vi "Periodic Tasks.vi"(8 "error in":errorcluster) -> ()   [LabVIEW 2016]
doc: "This VI runs in parallel to other tasks. It can contain as many user-defined periodic loops as you need. These can carry out PID or other sorts of timed response."
uses:
  Controls/Manual Shooter.ctl
  Controls/Shooter.ctl
  <vilib>/Rock Robotics/WPI/Solenoid/WPI_SolenoidValue.ctl
  <vilib>/Rock Robotics/WPI/DriverStation/WPI_DriverStationRobotMode2.ctl
  Controls/Auto Selector.ctl
  Controls/Gear Intake State.ctl
  Support Code/Change Detect.vi
  Support Code/Change Detect Boolean.vi
  <vilib>/Rock Robotics/WPI/Utilities/WPI_GetSetVariantRefNum.vi
  Robot Global Data.vi
  <vilib>/Rock Robotics/WPI/Solenoid/WPI_SolenoidSetEnum.vi
  <vilib>/Rock Robotics/Network Tables/NT Write Boolean.vi
  Controls/currentState.ctl
panel:
  in  "time to release(ms)":u32=800
  in  "Intake release speed":dbl=-0.5 format="%#_13g"
  in  "Intake gather speed":dbl=1.0 format="%#_13g"
  in  "Turret Deadband":dbl=0.5 format="%#_13g"
  out "Turret Stopped?":bool
  in  "turret error":dbl=4.0 format="%#_13g"
  in  "Turret Limit":dbl=90.0 format="%#_13g"
  out "low pass":dbl
  in  "auto gear on?":bool
  in  "turret reset":bool
  in  "Indexer % M":dbl=0.9 format="%#_13g"
  in  "M - Bot - Boiler":dbl=1450.0 format="%#_13g"
  in  "M - Top - Boiler":dbl=3950.0 format="%#_13g"
  in  "M - Bot - Airship":dbl=1500.0 format="%#_13g"
  in  "M - Top - Airship":dbl=4550.0 format="%#_13g"
  in  "autoGearRate":u32=10
  in  "Bot CPR":dbl=1024.0
  in  "Top CPR":dbl=1.0
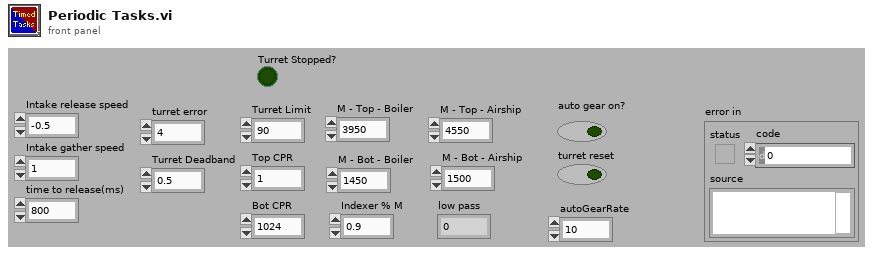
[diagram p1: front panel]
types:
  T1 = typedef "Shooter.ctl" = enum16{"Manual Control", "Get Setpoint", "Check Setpoint"}
  T2 = typedef "Manual Shooter.ctl" = enum16{"init", "Prepare - Airship", "Prepare - Boiler", "Burst mode"}
  T3 = typedef "WPI_RobotDriveDevRef.ctl" = cluster{"DevStatus":errorcluster, "Motors[]":T4[], "Square Inputs":bool, "Max Output":dbl}
  T4 = typedef "WPI_MotorControlDeviceRef.ctl" = cluster{"DeviceStatus":errorcluster, "Type":T5, "PWM":cluster{"PWM Channel":T6, "DeadBand":T7}, "CAN":cluster{"Device Number":u8, "SetOutput VI Ref":variant, "GetOutput VI Ref":variant, "Enable VI Ref":variant, "Disable VI Ref":variant, "Data":variant}, "Invert":bool}
  T5 = typedef "WPI_MotorControlType.ctl" = enum16{"PWM", "CAN"}
  T6 = typedef "FPGA_DIOPWMChannel.ctl" = enum8{"PWM 0", "PWM 1", "PWM 2", "PWM 3", "PWM 4", "PWM 5", "PWM 6", "PWM 7", "PWM 8", "PWM 9", "PWM MXP 0", "PWM MXP 1", "PWM MXP 2", "PWM MXP 3", "PWM MXP 4", "PWM MXP 5", "PWM MXP 6", "PWM MXP 7", "PWM MXP 8", "PWM MXP 9", "Invalid"}
  T7 = typedef "WPI_PWMDeadband.ctl" = cluster{"Name":string, "maxPositivePwm":i32, "minPositivePwm":i32, "centerPwm":i32, "maxNegativePwm":i32, "minNegativePwm":i32, "angularRange":u16}
  T8 = typedef "WPI_SolenoidDevRef.ctl" = cluster{"DevStatus":errorcluster, "Pneumatics Control Module":u8, "Forward Solenoid Channel":T9, "Reverse Solenoid Channel":T9}
  T9 = typedef "WPI_SolenoidChannel.ctl" = enum8{"Solenoid 0", "Solenoid 1", "Solenoid 2", "Solenoid 3", "Solenoid 4", "Solenoid 5", "Solenoid 6", "Solenoid 7", "Invalid"}
  T10 = cluster{"positions[0]":cluster{"x":i32, "y":i32}, "positions[1]":cluster{"x":i32, "y":i32}, "positions[2]":cluster{"x":i32, "y":i32}, "positions[3]":cluster{"x":i32, "y":i32}, "positions[4]":cluster{"x":i32, "y":i32}, "positions[5]":cluster{"x":i32, "y":i32}, "positions[6]":cluster{"x":i32, "y":i32}, "positions[7]":cluster{"x":i32, "y":i32}, "positions[8]":cluster{"x":i32, "y":i32}}
  T11 = cluster{"Buttons[0]":bool, "Buttons[1]":bool, "Buttons[2]":bool, "Buttons[3]":bool, "Buttons[4]":bool, "Buttons[5]":bool, "Buttons[6]":bool, "Buttons[7]":bool, "Buttons[8]":bool}
  T12 = typedef "WPI_SolenoidValue.ctl" = enum16{"Off", "On", "Forward", "Reverse"}
  T13 = typedef "WPI_DriverStationRobotMode2.ctl" = enum16{"Autonomous Disabled", "Autonomous Enabled", "Teleop Disabled", "Teleop Enabled", "Disconnected", "Finish", "Test Disabled", "Test Enabled", "Emergency Stopped"}
  T14 = cluster{"Axes[0]":dbl, "Axes[1]":dbl, "Axes[2]":dbl, "Axes[3]":dbl, "Axes[4]":dbl, "Axes[5]":dbl, "Axes[6]":dbl, "Axes[7]":dbl, "Axes[8]":dbl}
  T15 = typedef "Gear Intake State.ctl" = enum16{"init", "Gather", "Release"}
  T16 = typedef "WPI_DigitalInputDevRef.ctl" = cluster{"DevStatus":errorcluster, "DIO Channel":T17}
  T17 = typedef "FPGA_DIOChannel.ctl" = enum8{"DIO 0", "DIO 1", "DIO 2", "DIO 3", "DIO 4", "DIO 5", "DIO 6", "DIO 7", "DIO 8", "DIO 9", "DIO MXP 0", "DIO MXP 1", "DIO MXP 2", "DIO MXP 3", "DIO MXP 4", "DIO MXP 5", "DIO MXP 6", "DIO MXP 7", "DIO MXP 8", "DIO MXP 9", "DIO MXP 10", "DIO MXP 11", "DIO MXP 12", "DIO MXP 13", "DIO MXP 14", "DIO MXP 15", "SPI Port CS1", "SPI Port CS2", "SPI Port CS3", "SPI Port MISO", "SPI Port MOSI", "Invalid"}
  T18 = typedef "Auto Selector.ctl" = enum16{"Gear + Fuel with Vision", "Gear + Fuel no Vision", "Middle Gear", "Gear - Feeder peg", "Nothing"}
  T19 = cluster{"Top":bool, "Left":bool, "Right":bool, "Bottom":bool}
  T20 = typedef "currentState.ctl" = enum16{"init", "gearUp", "gearDown"}
  T21 = typedef "WPI_CounterDevRef.ctl" = cluster{"DevStatus":errorcluster, "CntIndex":T22}
  T22 = typedef "FPGA_CounterCtrSystemIndex.ctl" = enum8{"Ctr 0", "Ctr 1", "Ctr 2", "Ctr 3", "Ctr 4", "Ctr 5", "Ctr 6", "Ctr 7", "Invalid"}
  T23 = typedef "WPI_EncoderDevRef.ctl" = cluster{"DevStatus":errorcluster, "EncoderIndex":T24, "CounterIndex":T22, "DistancePerCount":dbl, "Decoding Type":T25}
  T24 = typedef "FPGA_EncoderIdx.ctl" = enum8{"Enc 0", "Enc 1", "Enc 2", "Enc 3", "Enc 4", "Enc 5", "Enc 6", "Enc 7", "Invalid"}
  T25 = typedef "WPI_EncoderType.ctl" = enum16{"1x", "2x", "4x"}
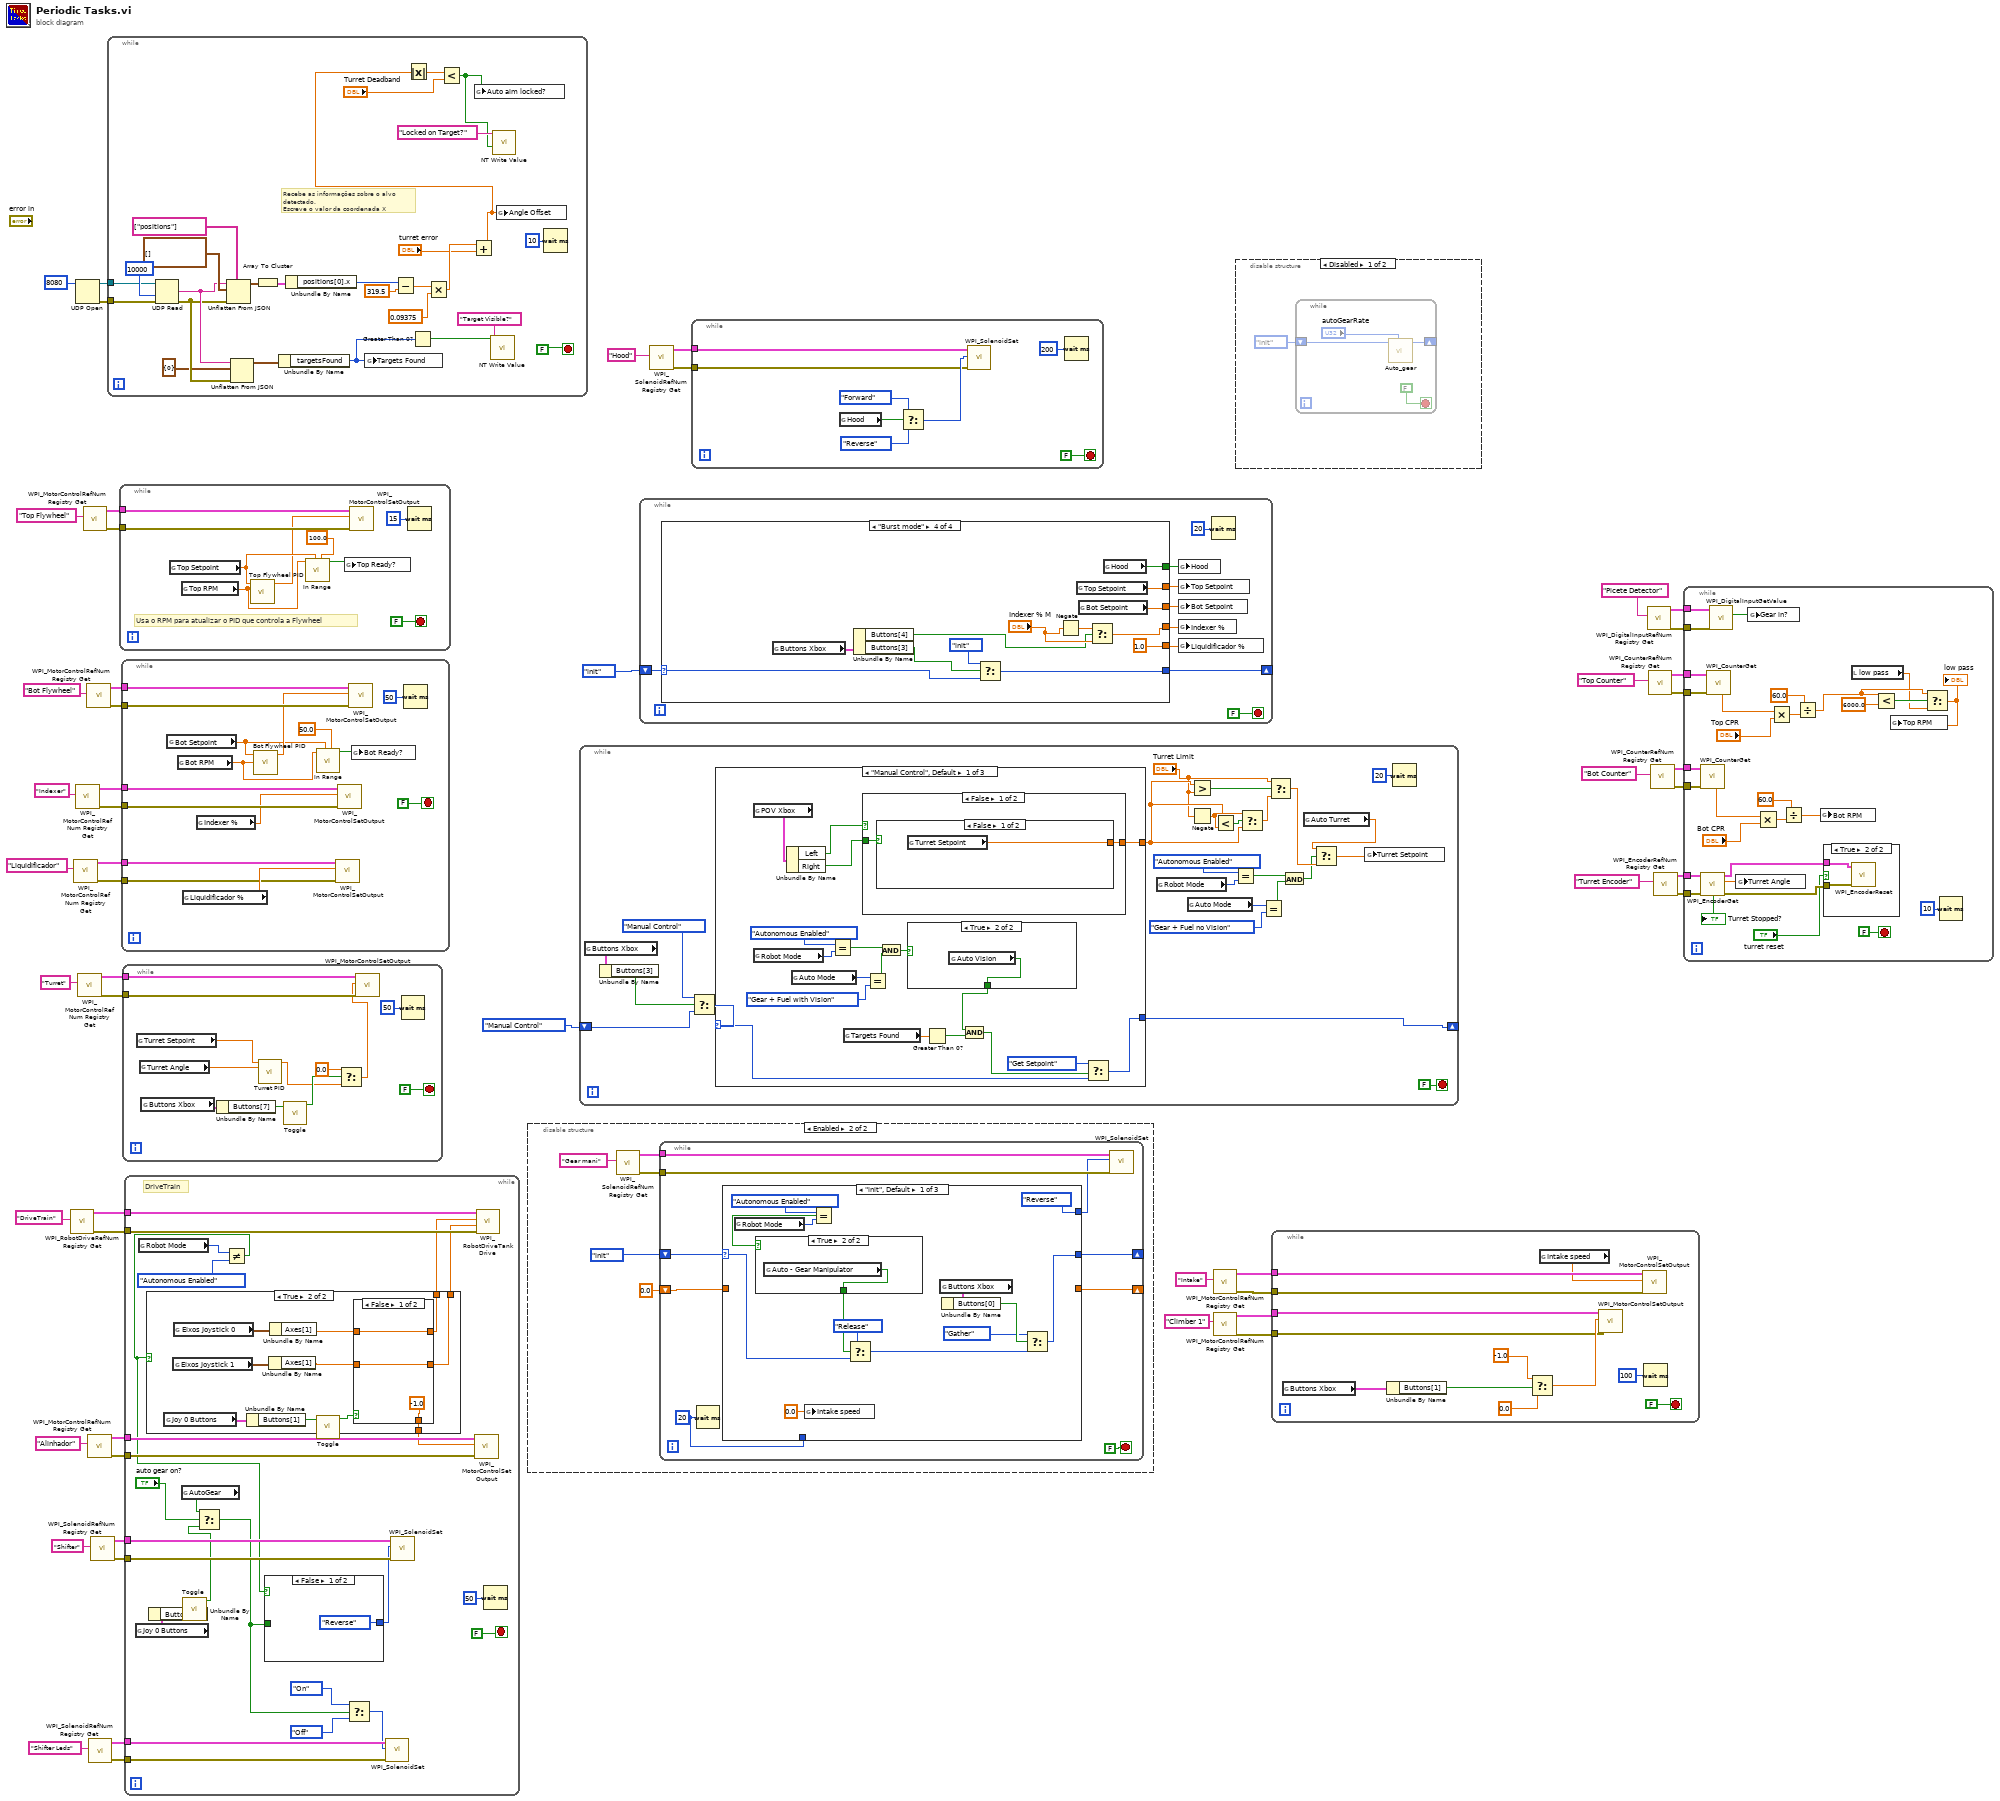
[diagram p0: block diagram]
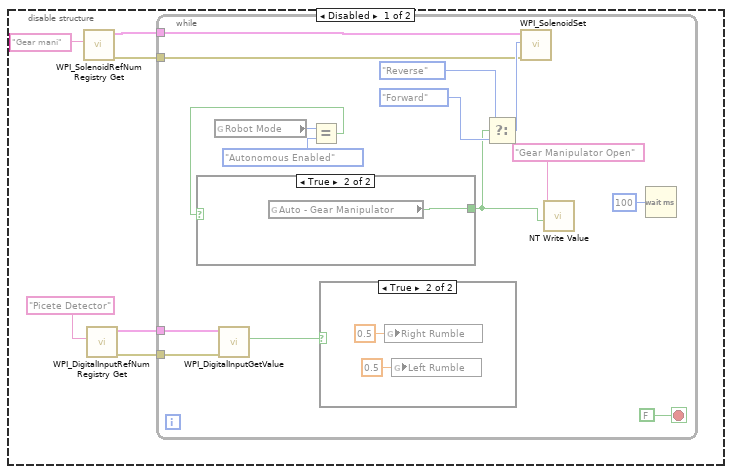
[diagram p2: hidden frame]
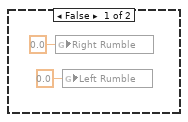
[diagram p3: hidden frame]
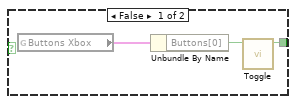
[diagram p4: hidden frame]
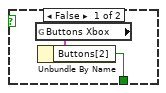
[diagram p5: hidden frame]
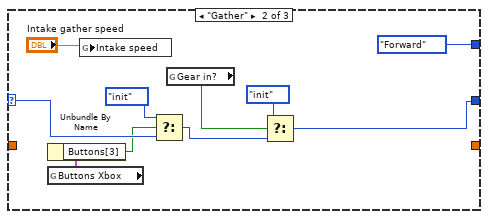
[diagram p6: hidden frame]
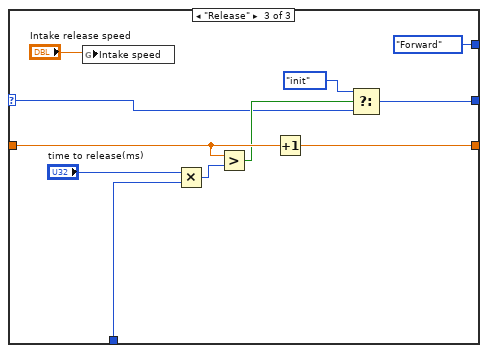
[diagram p7: hidden frame]
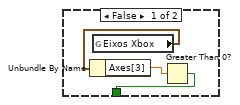
[diagram p9: hidden frame]
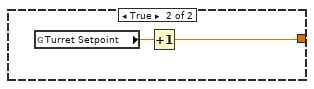
[diagram p10: hidden frame]
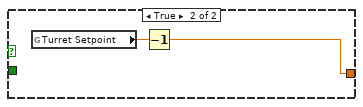
[diagram p11: hidden frame]
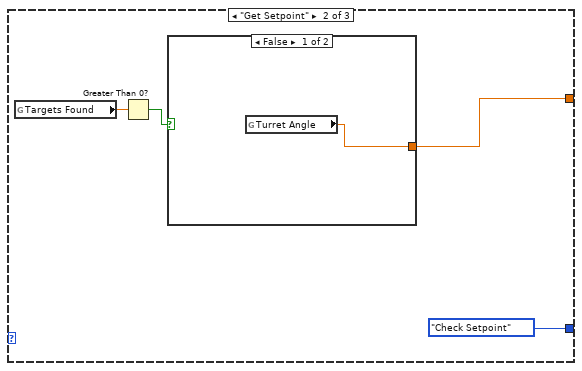
[diagram p12: hidden frame]
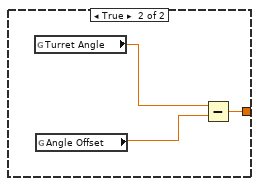
[diagram p13: hidden frame]
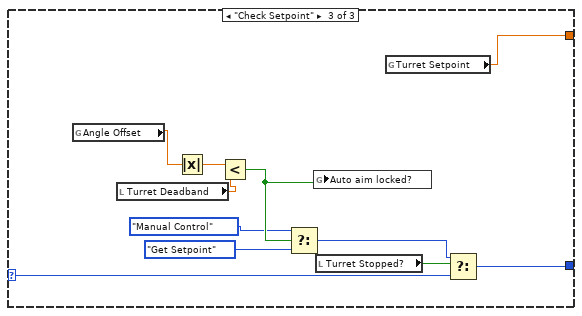
[diagram p14: hidden frame]
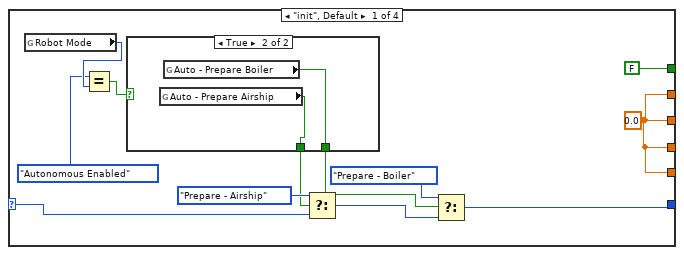
[diagram p15: hidden frame]
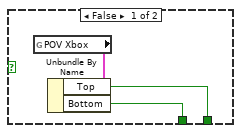
[diagram p16: hidden frame]
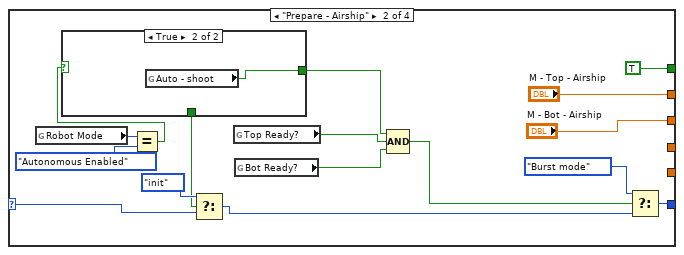
[diagram p17: hidden frame]
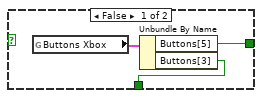
[diagram p18: hidden frame]
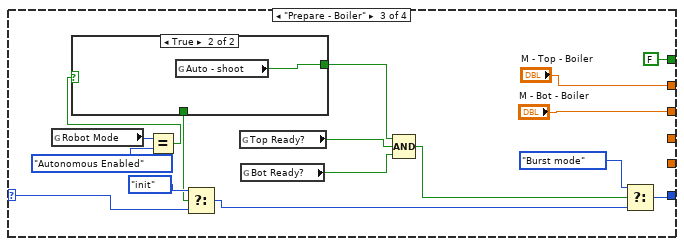
[diagram p19: hidden frame]
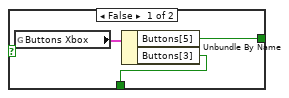
[diagram p20: hidden frame]
diagram:
  n1 = call <vilib>:"WPI_RobotDriveRefNum Registry Get.vi"("refnum name"="DriveTrain") -> ("error out"=w51:errorcluster, "RobotDriveDevRef"=w52:T3)  [unwired: 9 in]
  n2 = call <vilib>:"WPI_MotorControlRefNum Registry Get.vi"("refnum name"="Liquidificador") -> ("error out"=w27:errorcluster, "MotorControlDevRef"=w28:T4)  [unwired: 9 in]
  n3 = UDP Open(11:u16 8080 ("port")) -> (port=w5:refnum<k16>, 0:w6:errorcluster)  [unwired: 4 in, 1 out]
  n4 = call <vilib>:"WPI_MotorControlRefNum Registry Get.vi"("refnum name"="Indexer") -> ("error out"=w35:errorcluster, "MotorControlDevRef"=w34:T4)  [unwired: 9 in]
  n5 = call <vilib>:"WPI_MotorControlRefNum Registry Get.vi"("refnum name"="Turret") -> ("error out"=w36:errorcluster, "MotorControlDevRef"=w37:T4)  [unwired: 9 in]
  n6 = call <vilib>:"WPI_MotorControlRefNum Registry Get.vi"("refnum name"="Top Flywheel") -> ("error out"=w43:errorcluster, "MotorControlDevRef"=w44:T4)  [unwired: 9 in]
  n7 = call <vilib>:"WPI_MotorControlRefNum Registry Get.vi"("refnum name"="Bot Flywheel") -> ("error out"=w39:errorcluster, "MotorControlDevRef"=w40:T4)  [unwired: 9 in]
  n8 = call <vilib>:"WPI_MotorControlRefNum Registry Get.vi"("refnum name"="Alinhador") -> ("error out"=w15:errorcluster, "MotorControlDevRef"=w16:T4)  [unwired: 9 in]
  n9 = call <vilib>:"WPI_SolenoidRefNum Registry Get.vi"("refnum name"="Shifter Leds") -> ("error out"=w10:errorcluster, "SolenoidDevRef"=w9:T8)  [unwired: 9 in]
  n10 = call <vilib>:"WPI_SolenoidRefNum Registry Get.vi"("refnum name"="Shifter") -> ("error out"=w48:errorcluster, "SolenoidDevRef"=w49:T8)  [unwired: 9 in]
  n11 = while {
    tunnel: w6 -> [w76]
    tunnel: w5 -> [w75]
    stop <- FALSE stop-if-true
    # "Recebe as informações sobre o alvo detectado.\nEscreve o valor da coordenada X"
    n12 = UDP Read(connection ID=w75, timeout ms (25000)=10000, 8:w76) -> (data out=w66:string, error out=w65:errorcluster)  [unwired: 1 in, 3 out]
    n13 = Unflatten From JSON(path=string[] ["positions"], JSON string=w66, type and defaults=cluster{"x":i32, "y":i32}[] [] ("positions"), error in (no error)=w65) -> (value=w73:cluster{"x":i32, "y":i32}[])  [unwired: 3 in, 1 out]
    n14 = Unflatten From JSON(JSON string=w66, type and defaults=cluster{"targetsFound":i32} {"targetsFound"=0}, error in (no error)=w65) -> (value=w63:cluster{"targetsFound":i32})  [unwired: 4 in, 1 out]
    n15 = Array To Cluster(array=w73) -> (cluster=w72:T10)
    n16 = Unbundle By Name(w63) -> ("targetsFound"=w61:i32)
    n17 = Unbundle By Name(w72) -> ("positions[0].x"=w69:i32)
    n18 = global write "Robot Global Data.vi" "Targets Found"(w61) -> ()
    n19 = Subtract(x=w69, y=319.5) -> (x-y=w71:dbl)
    n20 = Greater Than 0?(x=w61) -> (x > 0?=w59:bool)
    n21 = Multiply(x=w71, y=0.09375) -> (x*y=w68:dbl)
    n22 = Add(x=w68, y="turret error") -> (x+y=w55:dbl)
    n23 = Absolute Value(x=w55) -> (abs(x)=w58:dbl)
    n24 = Less?(x=w58, y="Turret Deadband") -> (x < y?=w56:bool)
    n25 = global write "Robot Global Data.vi" "Auto aim locked?"(w56) -> ()
    n26 = call-poly <vilib>:"NT Write Value.vi"("Boolean"=w59, "Name"="Target Visible?") -> ()  [unwired: 9 in, 1 out]
    n27 = call-poly <vilib>:"NT Write Value.vi"("Boolean"=w56, "Name"="Locked on Target?") -> ()  [unwired: 9 in, 1 out]
    n28 = global write "Robot Global Data.vi" "Angle Offset"(w55) -> ()
    n29 = Wait (ms)(milliseconds to wait=u32 10) -> ()  [unwired: 1 out]
  }
  n30 = while {
    tunnel: w44 -> [w88]
    tunnel: w43 -> [w87]
    stop <- FALSE stop-if-true
    # "Usa o RPM para atualizar o PID que controla a Flywheel"
    n31 = global read "Robot Global Data.vi" "Top Setpoint"() -> (w83:dbl)
    n32 = global read "Robot Global Data.vi" "Top RPM"() -> (w84:dbl)
    n33 = call "Top Flywheel PID.vi"("Top RPM"=w84, "setpoint"=w83) -> ("output"=w81:dbl)  [unwired: 9 in]
    n34 = call "In Range.vi"("Range"=100.0, "Setpoint"=w83, "Value"=w84) -> ("in range?"=w85:bool)  [unwired: 8 in]
    n35 = global write "Robot Global Data.vi" "Top Ready?"(w85) -> ()
    n36 = call <vilib>:"WPI_MotorControlSetOutput.vi"("error in (no error)"=w87, "Output"=w81, "MotorControlDevRef"=w88) -> ()  [unwired: 6 in, 3 out]
    n37 = Wait (ms)(milliseconds to wait=u32 15) -> ()  [unwired: 1 out]
  }
  n38 = while {
    tunnel: w40 -> [w104]
    tunnel: w39 -> [w103]
    tunnel: w34 -> [w99]
    tunnel: w35 -> [w100]
    tunnel: w28 -> [w96]
    tunnel: w27 -> [w95]
    stop <- FALSE stop-if-true
    n39 = global read "Robot Global Data.vi" "Bot Setpoint"() -> (w90:dbl)
    n40 = global read "Robot Global Data.vi" "Bot RPM"() -> (w92:dbl)
    n41 = global read "Robot Global Data.vi" "Liquidificador %"() -> (w97:dbl)
    n42 = global read "Robot Global Data.vi" "Indexer %"() -> (w98:dbl)
    n43 = call "Bot Flywheel PID.vi"("Bot RPM"=w92, "setpoint"=w90) -> ("output"=w93:dbl)  [unwired: 9 in]
    n44 = call "In Range.vi"("Range"=50.0, "Setpoint"=w90, "Value"=w92) -> ("in range?"=w94:bool)  [unwired: 8 in]
    n45 = call <vilib>:"WPI_MotorControlSetOutput.vi"("error in (no error)"=w95, "Output"=w97, "MotorControlDevRef"=w96) -> ()  [unwired: 6 in, 3 out]
    n46 = call <vilib>:"WPI_MotorControlSetOutput.vi"("error in (no error)"=w100, "Output"=w98, "MotorControlDevRef"=w99) -> ()  [unwired: 6 in, 3 out]
    n47 = call <vilib>:"WPI_MotorControlSetOutput.vi"("error in (no error)"=w103, "Output"=w93, "MotorControlDevRef"=w104) -> ()  [unwired: 6 in, 3 out]
    n48 = global write "Robot Global Data.vi" "Bot Ready?"(w94) -> ()
    n49 = Wait (ms)(milliseconds to wait=u32 50) -> ()  [unwired: 1 out]
  }
  n50 = while {
    tunnel: w37 -> [w116]
    tunnel: w36 -> [w115]
    stop <- FALSE stop-if-true
    n51 = global read "Robot Global Data.vi" "Turret Setpoint"() -> (w111:dbl)
    n52 = global read "Robot Global Data.vi" "Turret Angle"() -> (w112:dbl)
    n53 = global read "Robot Global Data.vi" "Buttons Xbox"() -> (w110:T11)
    n54 = Unbundle By Name(w110) -> ("Buttons[7]"=w109:bool)
    n55 = call "Turret PID.vi"("setpoint"=w111, "Turret Angle"=w112) -> ("output"=w107:dbl)  [unwired: 13 in]
    n56 = call "Toggle.vi"("In"=w109) -> ("Toggled"=w108:bool)  [unwired: 10 in]
    n57 = Select(t=0.0, s=w108, f=w107) -> (s? t:f=w106:dbl)
    n58 = call <vilib>:"WPI_MotorControlSetOutput.vi"("error in (no error)"=w115, "Output"=w106, "MotorControlDevRef"=w116) -> ()  [unwired: 6 in, 3 out]
    n59 = Wait (ms)(milliseconds to wait=u32 50) -> ()  [unwired: 1 out]
  }
  n60 = while {
    tunnel: w52 -> [w140]
    tunnel: w51 -> [w139]
    tunnel: w49 -> [w138]
    tunnel: w48 -> [w137]
    tunnel: w16 -> [w127]
    tunnel: w15 -> [w126]
    tunnel: w10 -> [w123]
    tunnel: w9 -> [w122]
    stop <- FALSE stop-if-true
    # "DriveTrain"
    n61 = global read "Robot Global Data.vi" "Joy 0 Buttons"() -> (w134:T11)
    n62 = global read "Robot Global Data.vi" "Robot Mode"() -> (w131:T13)
    n63 = Unbundle By Name(w134) -> ("Buttons[0]"=w133:bool)
    n64 = global read "Robot Global Data.vi" "AutoGear"() -> (w135:bool)
    n65 = call "Toggle.vi"("In"=w133) -> ("Toggled"=w132:bool)  [unwired: 10 in]
    n66 = Select(t=w135, s="auto gear on?", f=w132) -> (s? t:f=w121:bool)
    n67 = Not Equal?(x=w131, y=WPI_DriverStationRobotMode2."Autonomous Enabled") -> (x != y?=w117:bool)
    n68 = case shown="True" w117 {
      tunnel: [w150 w160] -> w129
      tunnel: [w149 w159] -> w128
      tunnel: [-1.0 w155] -> w125
      frame False {
        n69 = global read "Robot Global Data.vi" "Auto Right Drive"() -> (w149:dbl)
        n70 = global read "Robot Global Data.vi" "Auto Left drive"() -> (w150:dbl)
      }
      frame True {
        n71 = global read "Robot Global Data.vi" "Joy 0 Buttons"() -> (w158:T11)
        n72 = global read "Robot Global Data.vi" "Eixos Joystick 1"() -> (w153:T14)
        n73 = global read "Robot Global Data.vi" "Eixos Joystick 0"() -> (w154:T14)
        n74 = Unbundle By Name(w158) -> ("Buttons[1]"=w156:bool)
        n75 = Unbundle By Name(w153) -> ("Axes[1]"=w151:dbl)
        n76 = Unbundle By Name(w154) -> ("Axes[1]"=w152:dbl)
        n77 = call "Toggle.vi"("In"=w156) -> ("Toggled"=w157:bool)  [unwired: 10 in]
        n78 = case shown="False" w157 {
          tunnel: w152 -> [w163 w165]
          tunnel: [w163 w167] -> w160
          tunnel: [w162 w166] -> w159
          tunnel: w151 -> [w162 w168]
          tunnel: [-1.0 1.0] -> w155
          frame False {
          }
          frame True {
            n79 = Negate(x=w165) -> (-x=w166:dbl)
            n80 = Negate(x=w168) -> (-x=w167:dbl)
          }
        }
      }
    }
    n81 = case shown="False" w117 {
      tunnel: [WPI_SolenoidValue."Reverse" ("Value") w145] -> w136
      tunnel: w121 -> [_ w144]
      frame False {
      }
      frame True {
        n82 = Select(t=WPI_SolenoidValue."Forward" ("Value"), s=w144, f=WPI_SolenoidValue."Reverse" ("Value")) -> (s? t:f=w145:T12)
      }
    }
    n83 = Select(t=WPI_SolenoidValue."On" ("Value"), s=w121, f=WPI_SolenoidValue."Off" ("Value")) -> (s? t:f=w120:T12)
    n84 = call-poly <vilib>:"WPI_SolenoidSet.vi"("error in (no error)"=w123, "Value"=w120, "SolenoidDevRef"=w122) -> ()  [unwired: 7 in, 2 out]
    n85 = call-poly <vilib>:"WPI_SolenoidSet.vi"("error in (no error)"=w137, "Value"=w136, "SolenoidDevRef"=w138) -> ()  [unwired: 7 in, 2 out]
    n86 = call <vilib>:"WPI_MotorControlSetOutput.vi"("error in (no error)"=w126, "Output"=w125, "MotorControlDevRef"=w127) -> ()  [unwired: 6 in, 3 out]
    n87 = call <vilib>:"WPI_RobotDriveTankDrive.vi"("error in (no error)"=w139, "Right axis value"=w128, "Left axis value"=w129, "RobotDriveDevRef"=w140) -> ()  [unwired: 5 in, 3 out]
    n88 = Wait (ms)(milliseconds to wait=u32 50) -> ()  [unwired: 1 out]
  }
  n89 = disable-structure shown="Enabled" {
    frame Disabled {
      n90 = call <vilib>:"WPI_SolenoidRefNum Registry Get.vi"("refnum name"="Gear mani") -> ("error out"=w173:errorcluster, "SolenoidDevRef"=w172:T8)  [unwired: 9 in]
      n91 = call <vilib>:"WPI_DigitalInputRefNum Registry Get.vi"("refnum name"="Picete Detector") -> ("error out"=w169:errorcluster, "DigitalInputDevRef"=w170:T16)  [unwired: 9 in]
      n92 = while {
        tunnel: w173 -> [w184]
        tunnel: w172 -> [w180]
        tunnel: w170 -> [w179]
        tunnel: w169 -> [w178]
        stop <- FALSE stop-if-true
        n93 = global read "Robot Global Data.vi" "Robot Mode"() -> (w183:T13)
        n94 = call <vilib>:"WPI_DigitalInputGetValue.vi"("error in (no error)"=w178, "DigitalInputDevRef"=w179) -> ("Value"=w177:bool)  [unwired: 7 in, 2 out]
        n95 = Equal?(x=w183, y=WPI_DriverStationRobotMode2."Autonomous Enabled") -> (x = y?=w181:bool)
        n96 = case shown="True" w181 {
          tunnel: [w194 w197] -> w175
          frame False {
            n97 = global read "Robot Global Data.vi" "Buttons Xbox"() -> (w196:T11)
            n98 = Unbundle By Name(w196) -> ("Buttons[0]"=w195:bool)
            n99 = call "Toggle.vi"("In"=w195) -> ("Toggled"=w194:bool)  [unwired: 10 in]
          }
          frame True {
            n100 = global read "Robot Global Data.vi" "Auto - Gear Manipulator"() -> (w197:bool)
          }
        }
        n101 = case shown="True" w177 {
          frame False {
            n102 = global write "Robot Global Data.vi" "Right Rumble"(0.0 ("Right Rumble")) -> ()
            n103 = global write "Robot Global Data.vi" "Left Rumble"(0.0 ("Left Rumble")) -> ()
          }
          frame True {
            n104 = global write "Robot Global Data.vi" "Right Rumble"(0.5 ("Right Rumble")) -> ()
            n105 = global write "Robot Global Data.vi" "Left Rumble"(0.5 ("Left Rumble")) -> ()
          }
        }
        n106 = Select(t=WPI_SolenoidValue."Reverse" ("Value"), s=w175, f=WPI_SolenoidValue."Forward" ("Value")) -> (s? t:f=w187:T12)
        n107 = call-poly <vilib>:"WPI_SolenoidSet.vi"("error in (no error)"=w184, "Value"=w187, "SolenoidDevRef"=w180) -> ()  [unwired: 7 in, 2 out]
        n108 = call-poly <vilib>:"NT Write Value.vi"("Boolean"=w175, "Name"="Gear Manipulator Open") -> ()  [unwired: 9 in, 1 out]
        n109 = Wait (ms)(milliseconds to wait=u32 100) -> ()  [unwired: 1 out]
      }
    }
    frame Enabled {
      n110 = call <vilib>:"WPI_SolenoidRefNum Registry Get.vi"("refnum name"="Gear mani") -> ("error out"=w199:errorcluster, "SolenoidDevRef"=w200:T8)  [unwired: 9 in]
      n111 = while {
        shift-right: [w207] -> _
        shift-left: Gear_Intake_State."init" -> [w211]
        tunnel: w200 -> [w209]
        tunnel: w199 -> [w208]
        shift-right: [w204] -> _
        shift-left: 0.0 -> [w205]
        stop <- FALSE stop-if-true
        w203 = u32 20 ("milliseconds to wait")
        n112 = Wait (ms)(milliseconds to wait=w203) -> ()  [unwired: 1 out]
        n113 = case shown="\"init\", Default" w211 {
          selector: w211 -> [w219 w231 w239]
          tunnel: [w222 w235 w246] -> w207
          tunnel: [WPI_SolenoidValue."Reverse" ("Value") WPI_SolenoidValue."Forward" ("Value") WPI_SolenoidValue."Forward" ("Value")] -> w206
          tunnel: w205 -> [_ _ w244]
          tunnel: [_ _ w245] -> w204
          tunnel: w203 -> [_ _ w242]
          frame "init", Default {
            n114 = global read "Robot Global Data.vi" "Robot Mode"() -> (w213:T13)
            n115 = global write "Robot Global Data.vi" "Intake speed"(0.0 ("Intake speed")) -> ()
            n116 = Equal?(x=WPI_DriverStationRobotMode2."Autonomous Enabled", y=w213) -> (x = y?=w212:bool)
            n117 = case shown="True" w212 {
              tunnel: [w225 w227] -> w218
              frame False {
                n118 = global read "Robot Global Data.vi" "Buttons Xbox"() -> (w226:T11)
                n119 = Unbundle By Name(w226) -> ("Buttons[2]"=w225:bool)
              }
              frame True {
                n120 = global read "Robot Global Data.vi" "Auto - Gear Manipulator"() -> (w227:bool)
              }
            }
            n121 = Select(t=Gear_Intake_State."Release", s=w218, f=w219) -> (s? t:f=w220:T15)
            n122 = global read "Robot Global Data.vi" "Buttons Xbox"() -> (w224:T11)
            n123 = Unbundle By Name(w224) -> ("Buttons[0]"=w223:bool)
            n124 = Select(t=Gear_Intake_State."Gather", s=w223, f=w220) -> (s? t:f=w222:T15)
          }
          frame "Gather" {
            n125 = global read "Robot Global Data.vi" "Buttons Xbox"() -> (w229:T11)
            n126 = Unbundle By Name(w229) -> ("Buttons[3]"=w228:bool)
            n127 = global write "Robot Global Data.vi" "Intake speed"("Intake gather speed") -> ()
            n128 = Select(t=Gear_Intake_State."init", s=w228, f=w231) -> (s? t:f=w232:T15)
            n129 = global read "Robot Global Data.vi" "Gear in?"() -> (w234:bool)
            n130 = Select(t=Gear_Intake_State."init", s=w234, f=w232) -> (s? t:f=w235:T15)
          }
          frame "Release" {
            n131 = global write "Robot Global Data.vi" "Intake speed"("Intake release speed") -> ()
            n132 = Multiply(x="time to release(ms)", y=w242) -> (x*y=w243:u32)
            n133 = Greater?(x=w244, y=w243) -> (0:w240:bool)
            n134 = Increment(x=w244) -> (x+1=w245:dbl)
            n135 = Select(t=Gear_Intake_State."init", s=w240, f=w239) -> (s? t:f=w246:T15)
          }
        }
        n136 = call-poly <vilib>:"WPI_SolenoidSet.vi"("error in (no error)"=w208, "Value"=w206, "SolenoidDevRef"=w209) -> ()  [unwired: 7 in, 2 out]
      }
    }
  }
  n137 = while {
    shift-right: [w260] -> _
    shift-left: Shooter."Manual Control" -> [w256]
    stop <- FALSE stop-if-true
    n138 = global read "Robot Global Data.vi" "Buttons Xbox"() -> (w259:T11)
    n139 = Unbundle By Name(w259) -> ("Buttons[3]"=w257:bool)
    n140 = Select(t=Shooter."Manual Control", s=w257, f=w256) -> (s? t:f=w258:T1)
    n141 = case shown="\"Manual Control\", Default" w258 {
      selector: w258 -> [w286 _ w315]
      tunnel: [w287 w305 w311] -> w268
      tunnel: [w285 Shooter."Check Setpoint" w318] -> w260
      frame "Manual Control", Default {
        n142 = global read "Robot Global Data.vi" "POV Xbox"() -> (w288:T19)
        n143 = global read "Robot Global Data.vi" "Robot Mode"() -> (w283:T13)
        n144 = Unbundle By Name(w288) -> ("Left"=w289:bool, "Right"=w290:bool)
        n145 = global read "Robot Global Data.vi" "Auto Mode"() -> (w281:T18)
        n146 = Equal?(x=WPI_DriverStationRobotMode2."Autonomous Enabled", y=w283) -> (x = y?=w282:bool)
        n147 = global read "Robot Global Data.vi" "Targets Found"() -> (w274:dbl)
        n148 = case shown="False" w289 {
          tunnel: w290 -> [w296 _]
          tunnel: [w295 w300] -> w287
          frame False {
            n149 = case shown="False" w296 {
              tunnel: [w297 w298] -> w295
              frame False {
                n150 = global read "Robot Global Data.vi" "Turret Setpoint"() -> (w297:dbl)
              }
              frame True {
                n151 = global read "Robot Global Data.vi" "Turret Setpoint"() -> (w299:dbl)
                n152 = Increment(x=w299) -> (x+1=w298:dbl)
              }
            }
          }
          frame True {
            n153 = global read "Robot Global Data.vi" "Turret Setpoint"() -> (w301:dbl)
            n154 = Decrement(x=w301) -> (x-1=w300:dbl)
          }
        }
        n155 = Equal?(x=w281, y=Auto_Selector."Gear + Fuel with Vision") -> (x = y?=w279:bool)
        n156 = And(x=w282, y=w279) -> (x .and. y?=w278:bool)
        n157 = case shown="True" w278 {
          tunnel: [w291 w294] -> w275
          frame False {
            n158 = global read "Robot Global Data.vi" "Eixos Xbox"() -> (w292:T14)
            n159 = Unbundle By Name(w292) -> ("Axes[3]"=w293:dbl)
            n160 = Greater Than 0?(x=w293) -> (x > 0?=w291:bool)
          }
          frame True {
            n161 = global read "Robot Global Data.vi" "Auto Vision"() -> (w294:bool)
          }
        }
        n162 = Greater Than 0?(x=w274) -> (x > 0?=w273:bool)
        n163 = And(x=w275, y=w273) -> (x .and. y?=w276:bool)
        n164 = Select(t=Shooter."Get Setpoint", s=w276, f=w286) -> (s? t:f=w285:T1)
      }
      frame "Get Setpoint" {
        n165 = global read "Robot Global Data.vi" "Targets Found"() -> (w303:dbl)
        n166 = Greater Than 0?(x=w303) -> (x > 0?=w302:bool)
        n167 = case shown="False" w302 {
          tunnel: [w306 w307] -> w305
          frame False {
            n168 = global read "Robot Global Data.vi" "Turret Angle"() -> (w306:dbl)
          }
          frame True {
            n169 = global read "Robot Global Data.vi" "Turret Angle"() -> (w309:dbl)
            n170 = global read "Robot Global Data.vi" "Angle Offset"() -> (w308:dbl)
            n171 = Subtract(x=w309, y=w308) -> (x-y=w307:dbl)
          }
        }
      }
      frame "Check Setpoint" {
        n172 = global read "Robot Global Data.vi" "Angle Offset"() -> (w320:dbl)
        n173 = local read "Turret Deadband"() -> (w310:dbl)
        n174 = Absolute Value(x=w320) -> (abs(x)=w319:dbl)
        n175 = Less?(x=w319, y=w310) -> (x < y?=w314:bool)
        n176 = Select(t=Shooter."Manual Control", s=w314, f=Shooter."Get Setpoint") -> (s? t:f=w316:T1)
        n177 = global write "Robot Global Data.vi" "Auto aim locked?"(w314) -> ()
        n178 = local read "Turret Stopped?"() -> (w317:bool)
        n179 = global read "Robot Global Data.vi" "Turret Setpoint"() -> (w311:dbl)
        n180 = Select(t=w316, s=w317, f=w315) -> (s? t:f=w318:T1)
      }
    }
    n181 = global read "Robot Global Data.vi" "Robot Mode"() -> (w263:T13)
    n182 = global read "Robot Global Data.vi" "Auto Mode"() -> (w252:T18)
    n183 = Greater?(x=w268, y="Turret Limit") -> (0:w265:bool)
    n184 = Negate(x="Turret Limit") -> (-x=w269:dbl)
    n185 = Less?(x=w268, y=w269) -> (x < y?=w270:bool)
    n186 = Equal?(x=WPI_DriverStationRobotMode2."Autonomous Enabled", y=w263) -> (x = y?=w253:bool)
    n187 = Select(t=w269, s=w270, f=w268) -> (s? t:f=w267:dbl)
    n188 = Equal?(x=w252, y=Auto_Selector."Gear + Fuel no Vision") -> (x = y?=w250:bool)
    n189 = Select(t="Turret Limit", s=w265, f=w267) -> (s? t:f=w262:dbl)
    n190 = And(x=w253, y=w250) -> (x .and. y?=w249:bool)
    n191 = global read "Robot Global Data.vi" "Auto Turret"() -> (w261:dbl)
    n192 = Select(t=w261, s=w249, f=w262) -> (s? t:f=w254:dbl)
    n193 = global write "Robot Global Data.vi" "Turret Setpoint"(w254) -> ()
    n194 = Wait (ms)(milliseconds to wait=u32 20) -> ()  [unwired: 1 out]
  }
  n195 = while {
    shift-right: [w325] -> _
    shift-left: Manual_Shooter."init" -> [w328]
    stop <- FALSE stop-if-true
    n196 = case shown="\"Burst mode\"" w328 {
      selector: w328 -> [w340 w357 w378 w395]
      tunnel: [FALSE TRUE FALSE w397] -> w327
      tunnel: [w333 "M - Bot - Airship" "M - Bot - Boiler" w398] -> w326
      tunnel: [w336 w359 w377 w396] -> w325
      tunnel: [w333 _ _ w391] -> w324
      tunnel: [w333 "M - Top - Airship" "M - Top - Boiler" w399] -> w323
      tunnel: [w333 _ _ 1.0 ("Liquidificador %")] -> w322
      frame "init", Default {
        w333 = 0.0
        n197 = global read "Robot Global Data.vi" "Robot Mode"() -> (w331:T13)
        n198 = Equal?(x=WPI_DriverStationRobotMode2."Autonomous Enabled", y=w331) -> (x = y?=w332:bool)
        n199 = case shown="True" w332 {
          tunnel: [w343 w345] -> w338
          tunnel: [w342 w346] -> w334
          frame False {
            n200 = global read "Robot Global Data.vi" "POV Xbox"() -> (w344:T19)
            n201 = Unbundle By Name(w344) -> ("Top"=w342:bool, "Bottom"=w343:bool)
          }
          frame True {
            n202 = global read "Robot Global Data.vi" "Auto - Prepare Airship"() -> (w345:bool)
            n203 = global read "Robot Global Data.vi" "Auto - Prepare Boiler"() -> (w346:bool)
          }
        }
        n204 = Select(t=Manual_Shooter."Prepare - Airship", s=w338, f=w340) -> (s? t:f=w337:T2)
        n205 = Select(t=Manual_Shooter."Prepare - Boiler", s=w334, f=w337) -> (s? t:f=w336:T2)
      }
      frame "Prepare - Airship" {
        n206 = global read "Robot Global Data.vi" "Robot Mode"() -> (w349:T13)
        n207 = Equal?(x=w349, y=WPI_DriverStationRobotMode2."Autonomous Enabled") -> (x = y?=w347:bool)
        n208 = case shown="True" w347 {
          tunnel: [w364 _] -> w354
          tunnel: [w363 w366] -> w351
          frame False {
            n209 = global read "Robot Global Data.vi" "Buttons Xbox"() -> (w365:T11)
            n210 = Unbundle By Name(w365) -> ("Buttons[5]"=w363:bool, "Buttons[3]"=w364:bool)
          }
          frame True {
            n211 = global read "Robot Global Data.vi" "Auto - shoot"() -> (w366:bool)
          }
        }
        n212 = Select(t=Manual_Shooter."init", s=w354, f=w357) -> (s? t:f=w356:T2)
        n213 = global read "Robot Global Data.vi" "Top Ready?"() -> (w353:bool)
        n214 = global read "Robot Global Data.vi" "Bot Ready?"() -> (w352:bool)
        n215 = Compound Arithmetic op=AND(w351, w353, w352) -> (w350:bool)
        n216 = Select(t=Manual_Shooter."Burst mode", s=w350, f=w356) -> (s? t:f=w359:T2)
      }
      frame "Prepare - Boiler" {
        n217 = global read "Robot Global Data.vi" "Robot Mode"() -> (w369:T13)
        n218 = Equal?(x=w369, y=WPI_DriverStationRobotMode2."Autonomous Enabled") -> (x = y?=w368:bool)
        n219 = case shown="True" w368 {
          tunnel: [w384 _] -> w379
          tunnel: [w383 w386] -> w373
          frame False {
            n220 = global read "Robot Global Data.vi" "Buttons Xbox"() -> (w385:T11)
            n221 = Unbundle By Name(w385) -> ("Buttons[5]"=w383:bool, "Buttons[3]"=w384:bool)
          }
          frame True {
            n222 = global read "Robot Global Data.vi" "Auto - shoot"() -> (w386:bool)
          }
        }
        n223 = Select(t=Manual_Shooter."init", s=w379, f=w378) -> (s? t:f=w381:T2)
        n224 = global read "Robot Global Data.vi" "Top Ready?"() -> (w371:bool)
        n225 = global read "Robot Global Data.vi" "Bot Ready?"() -> (w370:bool)
        n226 = Compound Arithmetic op=AND(w373, w371, w370) -> (w372:bool)
        n227 = Select(t=Manual_Shooter."Burst mode", s=w372, f=w381) -> (s? t:f=w377:T2)
      }
      frame "Burst mode" {
        n228 = global read "Robot Global Data.vi" "Buttons Xbox"() -> (w394:T11)
        n229 = Unbundle By Name(w394) -> ("Buttons[4]"=w388:bool, "Buttons[3]"=w393:bool)
        n230 = Select(t=Manual_Shooter."init", s=w393, f=w395) -> (s? t:f=w396:T2)
        n231 = Negate(x="Indexer % M") -> (-x=w390:dbl)
        n232 = global read "Robot Global Data.vi" "Top Setpoint"() -> (w399:dbl)
        n233 = global read "Robot Global Data.vi" "Bot Setpoint"() -> (w398:dbl)
        n234 = Select(t=w390, s=w388, f="Indexer % M") -> (s? t:f=w391:dbl)
        n235 = global read "Robot Global Data.vi" "Hood"() -> (w397:bool)
      }
    }
    n236 = global write "Robot Global Data.vi" "Hood"(w327) -> ()
    n237 = global write "Robot Global Data.vi" "Top Setpoint"(w323) -> ()
    n238 = global write "Robot Global Data.vi" "Bot Setpoint"(w326) -> ()
    n239 = global write "Robot Global Data.vi" "Indexer %"(w324) -> ()
    n240 = global write "Robot Global Data.vi" "Liquidificador %"(w322) -> ()
    n241 = Wait (ms)(milliseconds to wait=u32 20) -> ()  [unwired: 1 out]
  }
  n242 = call <vilib>:"WPI_SolenoidRefNum Registry Get.vi"("refnum name"="Hood") -> ("error out"=w30:errorcluster, "SolenoidDevRef"=w31:T8)  [unwired: 9 in]
  n243 = while {
    tunnel: w31 -> [w402]
    tunnel: w30 -> [w401]
    stop <- FALSE stop-if-true
    n244 = global read "Robot Global Data.vi" "Hood"() -> (w400:bool)
    n245 = Select(t=WPI_SolenoidValue."Forward" ("Value"), s=w400, f=WPI_SolenoidValue."Reverse" ("Value")) -> (s? t:f=w405:T12)
    n246 = call-poly <vilib>:"WPI_SolenoidSet.vi"("error in (no error)"=w401, "Value"=w405, "SolenoidDevRef"=w402) -> ()  [unwired: 7 in, 2 out]
    n247 = Wait (ms)(milliseconds to wait=u32 200) -> ()  [unwired: 1 out]
  }
  n248 = call <vilib>:"WPI_MotorControlRefNum Registry Get.vi"("refnum name"="Intake") -> ("error out"=w12:errorcluster, "MotorControlDevRef"=w13:T4)  [unwired: 9 in]
  n249 = call <vilib>:"WPI_MotorControlRefNum Registry Get.vi"("refnum name"="Climber 1") -> ("error out"=w46:errorcluster, "MotorControlDevRef"=w47:T4)  [unwired: 9 in]
  n250 = disable-structure shown="Disabled" {
    frame Disabled {
      n251 = while {
        shift-right: [w409] -> _
        shift-left: currentState."init" -> [w411]
        stop <- FALSE stop-if-true
        n252 = call "Auto_gear.vi"("autoGearRate"="autoGearRate", "Enum in"=w411) -> ("Enum out"=w409:T20)  [unwired: 9 in]
      }
    }
    frame Enabled {
    }
  }
  n253 = while {
    tunnel: w47 -> [w419]
    tunnel: w46 -> [w418]
    tunnel: w13 -> [w415]
    tunnel: w12 -> [w414]
    stop <- FALSE stop-if-true
    n254 = global read "Robot Global Data.vi" "Buttons Xbox"() -> (w424:T11)
    n255 = Unbundle By Name(w424) -> ("Buttons[1]"=w423:bool)
    n256 = Select(t=-1.0, s=w423, f=0.0) -> (s? t:f=w420:dbl)
    n257 = global read "Robot Global Data.vi" "Intake speed"() -> (w413:dbl)
    n258 = call <vilib>:"WPI_MotorControlSetOutput.vi"("error in (no error)"=w418, "Output"=w420, "MotorControlDevRef"=w419) -> ()  [unwired: 6 in, 3 out]
    n259 = call <vilib>:"WPI_MotorControlSetOutput.vi"("error in (no error)"=w414, "Output"=w413, "MotorControlDevRef"=w415) -> ()  [unwired: 6 in, 3 out]
    n260 = Wait (ms)(milliseconds to wait=u32 100) -> ()  [unwired: 1 out]
  }
  n261 = call <vilib>:"WPI_DigitalInputRefNum Registry Get.vi"("refnum name"="Picete Detector") -> ("error out"=w1:errorcluster, "DigitalInputDevRef"=w2:T16)  [unwired: 9 in]
  n262 = call <vilib>:"WPI_CounterRefNum Registry Get.vi"("refnum name"="Top Counter") -> ("error out"=w20:errorcluster, "CounterDevRef"=w18:T21)  [unwired: 9 in]
  n263 = call <vilib>:"WPI_CounterRefNum Registry Get.vi"("refnum name"="Bot Counter") -> ("error out"=w21:errorcluster, "CounterDevRef"=w23:T21)  [unwired: 9 in]
  n264 = call <vilib>:"WPI_EncoderRefNum Registry Get.vi"("refnum name"="Turret Encoder") -> ("error out"=w25:errorcluster, "EncoderDevRef"=w24:T23)  [unwired: 9 in]
  n265 = while {
    tunnel: w18 -> [w454]
    tunnel: w20 -> [w453]
    tunnel: w23 -> [w442]
    tunnel: w21 -> [w443]
    tunnel: w24 -> [w441]
    tunnel: w25 -> [w440]
    tunnel: w2 -> [w427]
    tunnel: w1 -> [w426]
    stop <- FALSE stop-if-true
    n266 = call <vilib>:"WPI_CounterGet.vi"("error in (no error)"=w443, "CounterDevRef in"=w442) -> ("Period (sec)"=w446:dbl)  [unwired: 4 in, 5 out]
    n267 = call <vilib>:"WPI_EncoderGet.vi"("error in (no error)"=w440, "EncoderDevRef"=w441) -> ("error out"=w437:errorcluster, "Distance"=w439:dbl, "EncoderDevRef"=w438:T23, "Stopped"=→"Turret Stopped?":bool)  [unwired: 4 in, 2 out]
    n268 = call <vilib>:"WPI_CounterGet.vi"("error in (no error)"=w453, "CounterDevRef in"=w454) -> ("Period (sec)"=w434:dbl)  [unwired: 4 in, 5 out]
    n269 = call <vilib>:"WPI_DigitalInputGetValue.vi"("error in (no error)"=w426, "DigitalInputDevRef"=w427) -> ("Value"=w425:bool)  [unwired: 7 in, 2 out]
    n270 = global write "Robot Global Data.vi" "Turret Angle"(w439) -> ()
    n271 = global write "Robot Global Data.vi" "Gear in?"(w425) -> ()
    n272 = Multiply(x=w446, y="Bot CPR") -> (x*y=w444:dbl)
    n273 = Multiply(x=w434, y="Top CPR") -> (x*y=w452:dbl)
    n274 = Divide(x=60.0, y=w444) -> (x/y=w448:dbl)
    n275 = Divide(x=60.0, y=w452) -> (x/y=w433:dbl)
    n276 = global write "Robot Global Data.vi" "Bot RPM"(w448) -> ()
    n277 = case shown="True" "turret reset" {
      tunnel: w438 -> [_ w456]
      tunnel: w437 -> [_ w455]
      frame False {
      }
      frame True {
        n278 = call <vilib>:"WPI_EncoderReset.vi"("error in (no error)"=w455, "EncoderDevRef"=w456) -> ()  [unwired: 8 in, 2 out]
      }
    }
    n279 = local read "low pass"() -> (w429:dbl)
    n280 = Less?(x=w433, y=6000.0) -> (x < y?=w430:bool)
    n281 = Select(t=w433, s=w430, f=w429) -> (s? t:f=w432:dbl)
    "low pass" <- w432
    n282 = global write "Robot Global Data.vi" "Top RPM"(w432) -> ()
    n283 = Wait (ms)(milliseconds to wait=u32 10) -> ()  [unwired: 1 out]
  }
